vi "Write Structure.vi"(8 "error in (no error)":errorcluster, 10 "Structure.lvclass":refnum<class "Structure.lvclass">, 11 "ParseGDSII in":refnum<class "ParseGDSII.lvclass">) -> (0 "error out":errorcluster, 3 "ParseGDSII out":refnum<class "ParseGDSII.lvclass">)   [LabVIEW 2019, in "ParseGDSII.lvclass"]
uses:
  ParseGDSII.lvclass
  Structures/Structure.lvclass
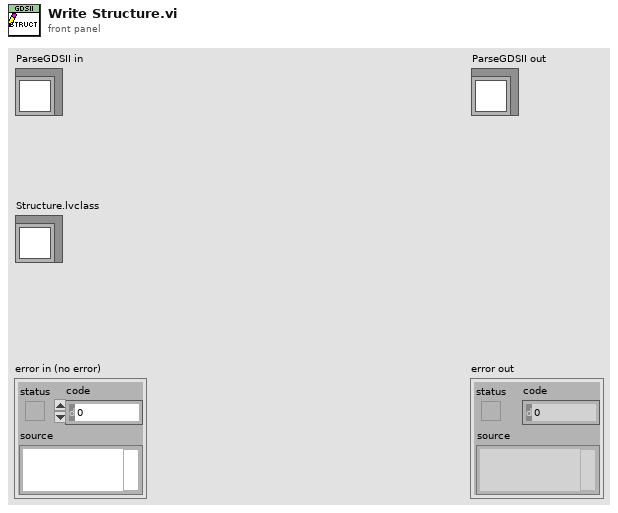
[diagram p1: front panel]
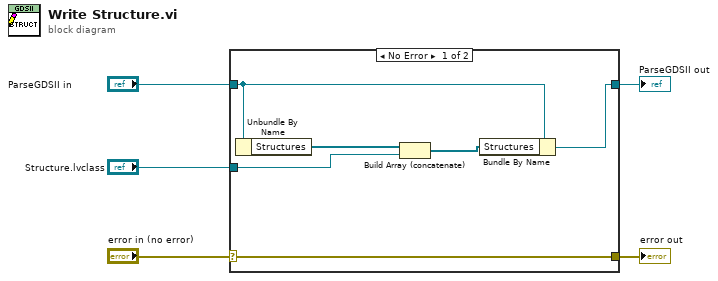
[diagram p0: block diagram]
diagram:
  n1 = case shown="No Error" "error in (no error)" {
    selector: "error in (no error)" -> [w11 w12]
    tunnel: [w11 w12] -> w4
    tunnel: [w10 w13] -> w2
    tunnel: "ParseGDSII in" -> [w9 w13]
    tunnel: "Structure.lvclass" -> [w6 _]
    frame No Error {
      n2 = Unbundle By Name(w9) -> ("Structures"=w8:refnum<class "Structure.lvclass">[])
      n3 = Build Array (concatenate)(w8, w6) -> (w7:refnum<class "Structure.lvclass">[])
      n4 = Bundle By Name(cluster=w9, "Structures"=w7) -> (w10:refnum<class "ParseGDSII.lvclass">)
    }
    frame Error {
    }
  }
  "error out" <- w4
  "ParseGDSII out" <- w2
